vi "SetTxFrequency.vi"(6 "Legacy (f)?":bool, 8 "error in (no error)":errorcluster, 10 "TxFrequencies":dbl[](array[numeric]) format="%.2f") -> (0 "error out":errorcluster)   [LabVIEW 2011]
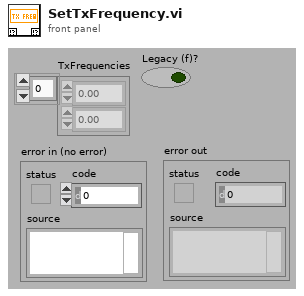
[diagram p1: front panel]
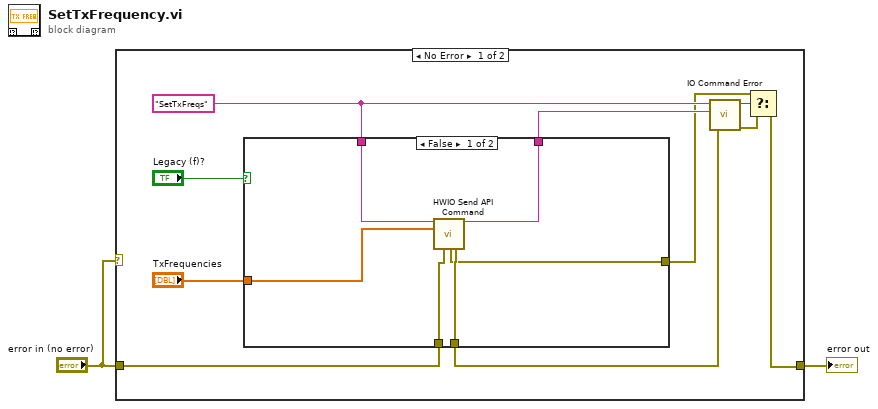
[diagram p0: block diagram]
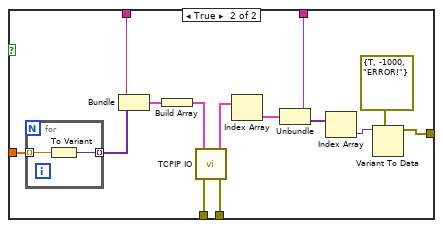
[diagram p2: hidden frame]
diagram:
  n1 = case shown="No Error" "error in (no error)" {
    tunnel: "error in (no error)" -> [w11 w35]
    tunnel: [w5 w35] -> w2
    frame No Error {
      w9 = "SetTxFreqs"
      n2 = case shown="False" "Legacy (f)?" {
        tunnel: "TxFrequencies" -> [w15 w32]
        tunnel: w11 -> [w14 w30]
        tunnel: [w18 w28] -> w10
        tunnel: w9 -> [w16 w27]
        tunnel: [w17 w23] -> w8
        tunnel: [w13 w19] -> w4
        frame False {
          n3 = call "HWIO Send API Command.vi"("Action"=w16, "Double"=w15, "error in (no error)"=w14) -> ("Action out"=w17:string, "HWError"=w13:errorcluster, "error out"=w18:errorcluster)  [unwired: 5 in, 5 out]
        }
        frame True {
          n4 = for {
            tunnel: w32 -> [w34] mode=indexing
            tunnel: [w33] -> w31 mode=indexing
            n5 = To Variant(anything=w34) -> (Variant=w33:variant)
          }
          n6 = Bundle(w27, w31) -> (w29:cluster{string, variant[]})  [unwired: 1 out]
          n7 = Build Array(w29) -> (w26:cluster{string, variant[]}[])
          n8 = call "TCPIP IO.vi"("error in (no error)"=w30, "Commands"=w26) -> ("error out"=w28:errorcluster, "Responses"=w24:cluster{string, variant[]}[])  [unwired: 1 in, 3 out]
          n9 = Index Array(array=w24) -> (element=w25:cluster{string, variant[]})  [unwired: 1 in]
          n10 = Unbundle(w25) -> (w23:string, w20:variant[])
          n11 = Index Array(array=w20) -> (element=w22:variant)  [unwired: 1 in]
          n12 = Variant To Data(type=errorcluster {"status"=TRUE, "code"=-1000, "source"="ERROR!"} ("error out"), Variant=w22) -> (data=w19:errorcluster)  [unwired: 1 in, 1 out]
        }
      }
      n13 = call "IO Command Error.vi"("error in (no error)"=w10, "Command Returned (\"\")"=w8, "Command Sent (\"\")"=w9) -> ("error out"=w6:errorcluster, "HW ERR?"=w7:bool)  [unwired: 3 out]
      n14 = Select(t=w4, s=w7, f=w6) -> (s? t:f=w5:errorcluster)
    }
    frame Error {
    }
  }
  "error out" <- w2
